vi "XYZ stage tester.vi"() -> ()   [LabVIEW 2017]
uses:
  Global Variables/General Globals.vi
panel:
  in  "Open":bool
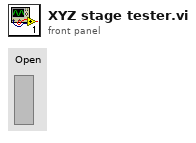
[diagram p1: front panel]
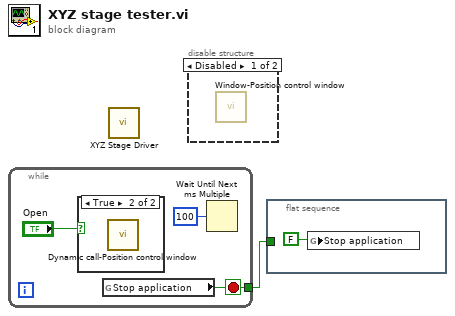
[diagram p0: block diagram]
diagram:
  n1 = while {
    tunnel: [w2] -> w1
    stop <- w2 stop-if-true
    n2 = case shown="True" "Open" {
      frame False {
      }
      frame True {
        n3 = call "Dynamic call-Position control window.vi"() -> ()  [unwired: 11 in, 1 out]
      }
    }
    n4 = global read "General Globals.vi" "Stop application"() -> (w2:bool)
    n5 = Wait Until Next ms Multiple(millisecond multiple=u32 100) -> ()  [unwired: 1 out]
  }
  n6 = call "XYZ Stage Driver.vi"() -> ()  [unwired: 11 in, 1 out]
  n7 = disable-structure shown="Disabled" {
    frame Disabled {
      n8 = call "Window-Position control window.vi"() -> ()  [unwired: 12 in]
    }
    frame Enabled {
    }
  }
  n9 = flat-sequence {
    tunnel: w1 -> [_]
    frame #0 {
      n10 = global write "General Globals.vi" "Stop application"(FALSE ("Stop application")) -> ()
    }
  }
